vi "getconfigtest.vi"() -> ()   [LabVIEW 2017, in "Gantry.lvclass"]
uses:
  Gantry.lvclass
  Type Definitions/Virtual Modes.ctl
  FlexWorktable/FlexWorktable.lvclass
panel:
  out "Active Config":string
  out "homed? 2":bool
  out "homed?":bool
  out "error out":errorcluster
  in  "Config Folder":path=path "C:/Users/husker/Desktop/gantry/Config"
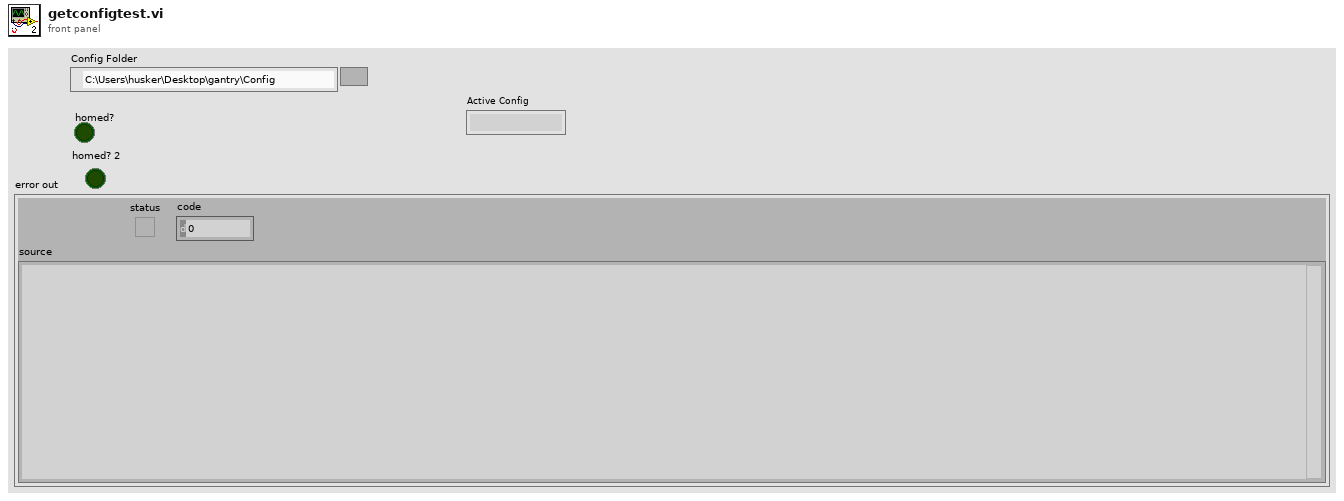
[diagram p1: front panel]
types:
  T1 = typedef "Virtual Modes.ctl" = enum16{"Nonvirtual", "Virtual"}
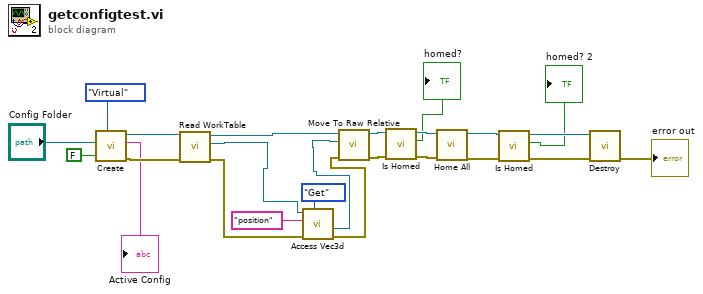
[diagram p0: block diagram]
diagram:
  n1 = call "Create.vi"("Virtual Mode"=Virtual_Modes."Virtual", "HOME?"=FALSE, "Config Folder"="Config Folder") -> ("error out"=w11:errorcluster, "Active Config"=→"Active Config":string, "Gantry out"=w10:refnum<class "Gantry.lvclass">)  [unwired: 6 in]
  n2 = call-dynamic "Read WorkTable.vi"("error in"=w11, "Gantry Class in"=w10) -> ("error out"=w7:errorcluster, "Worktable"=w5:refnum<class "FlexWorktable.lvclass">, "Gantry Class out"=w12:refnum<class "Gantry.lvclass">)  [unwired: 7 in]
  n3 = call-dynamic "Access Vec3d.vi"("Get/Set"=enum16{"Get", "Set"}."Get", "error in (no error)"=w7, "Key"="position", "FlexWorktable in"=w5) -> ("error out"=w4:errorcluster, "Value out"=w3:refnum<class "Vec3d.lvclass">)  [unwired: 5 in, 1 out]
  n4 = call-dynamic "Move To Raw Relative.vi"("error in"=w4, "Delta"=w3, "Gantry in"=w12) -> ("error out"=w15:errorcluster, "Gantry out"=w16:refnum<class "Gantry.lvclass">)  [unwired: 7 in]
  n5 = call "Is Homed.vi"("error in (no error)"=w15, "Gantry in"=w16) -> ("error out"=w13:errorcluster, "homed?"=→"homed?":bool, "Gantry out"=w18:refnum<class "Gantry.lvclass">)  [unwired: 7 in]
  n6 = call "Home All.vi"("error in (no error)"=w13, "Gantry in"=w18) -> ("error out"=w20:errorcluster, "Gantry out"=w22:refnum<class "Gantry.lvclass">)  [unwired: 8 in]
  n7 = call "Is Homed.vi"("error in (no error)"=w20, "Gantry in"=w22) -> ("error out"=w19:errorcluster, "homed?"=→"homed? 2":bool, "Gantry out"=w21:refnum<class "Gantry.lvclass">)  [unwired: 7 in]
  n8 = call "Destroy.vi"("error in"=w19, "Gantry Class in"=w21) -> ("error out"=→"error out":errorcluster)  [unwired: 9 in]
